vi "LINC Register Commit.vi"(4 "override? registration":bool, 8 "error in (no error)":errorcluster, 10 "register":T1={"COSMOS cmds (T)"=TRUE, "common cmds (T)"=TRUE, "handshake tlm (T)"=TRUE, "error tlm (T)"=TRUE}, 11 "LINC session":refnum<class "LINC.lvclass">) -> (0 "error out":errorcluster, 3 "dup LINC session":refnum<class "LINC.lvclass">)   [LabVIEW 2018, in "STEPkgDriver_LINC.lvlib" / "LINC.lvclass"]
uses:
  LINC.lvclass
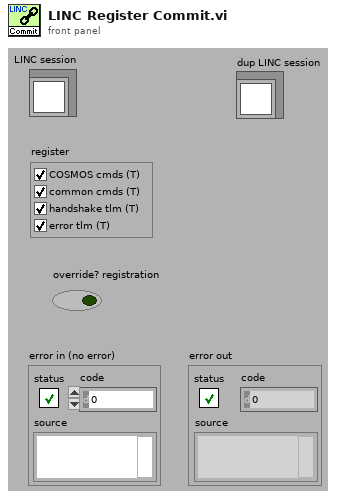
[diagram p1: front panel]
types:
  T1 = cluster{"COSMOS cmds (T)":bool, "common cmds (T)":bool, "handshake tlm (T)":bool, "error tlm (T)":bool}
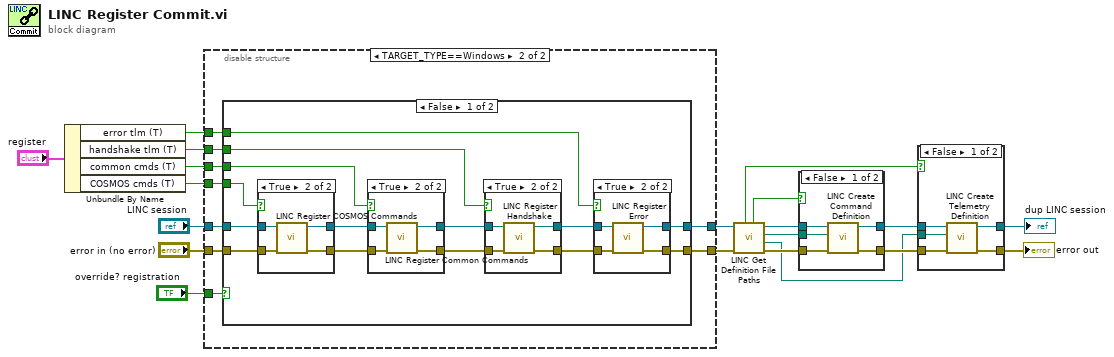
[diagram p0: block diagram]
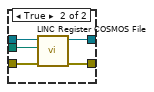
[diagram p8: hidden frame]
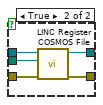
[diagram p9: hidden frame]
diagram:
  n1 = Unbundle By Name("register") -> ("error tlm (T)"=w5:bool, "handshake tlm (T)"=w2:bool, "common cmds (T)"=w3:bool, "COSMOS cmds (T)"=w4:bool)
  n2 = disable-structure shown="TARGET_TYPE==Windows" {
    disable-tunnel: "error in (no error)" -> [w21 w30]
    disable-tunnel: "LINC session" -> [w22 w29]
    disable-tunnel: [w21 w24] -> w16
    disable-tunnel: [w22 w25] -> w7
    disable-tunnel: w3 -> [_ w31]
    disable-tunnel: w5 -> [_ w26]
    disable-tunnel: w4 -> [_ w28]
    disable-tunnel: w2 -> [_ w27]
    disable-tunnel: "override? registration" -> [_ w23]
    frame condition #0 {
      # "Dynamic Registration is not available in any target type but Windows"
    }
    frame condition #1 (active) {
      n3 = case shown="False" w23 {
        tunnel: w31 -> [w45 _]
        tunnel: w30 -> [w44 w70]
        tunnel: w29 -> [w43 w71]
        tunnel: w28 -> [w40 _]
        tunnel: w27 -> [w37 _]
        tunnel: w26 -> [w34 _]
        tunnel: [w33 w71] -> w25
        tunnel: [w32 w70] -> w24
        frame False {
          n4 = case shown="True" w40 {
            tunnel: w44 -> [w58 w63]
            tunnel: w43 -> [w59 w62]
            tunnel: [w58 w61] -> w41
            tunnel: [w59 w60] -> w42
            frame False {
            }
            frame True {
              n5 = call "LINC Register COSMOS Commands.vi"("error in"=w63, "LINC session"=w62) -> ("error out"=w61:errorcluster, "dup LINC session"=w60:refnum<class "LINC.lvclass">)  [unwired: 8 in]
            }
          }
          n6 = case shown="True" w45 {
            tunnel: w41 -> [w65 w69]
            tunnel: [w65 w68] -> w38
            tunnel: [w64 w67] -> w39
            tunnel: w42 -> [w64 w66]
            frame False {
            }
            frame True {
              n7 = call "LINC Register Common Commands.vi"("error in"=w69, "LINC session"=w66) -> ("error out"=w68:errorcluster, "dup LINC session"=w67:refnum<class "LINC.lvclass">)  [unwired: 8 in]
            }
          }
          n8 = case shown="True" w37 {
            tunnel: w38 -> [w53 w57]
            tunnel: [w53 w56] -> w36
            tunnel: [w52 w55] -> w35
            tunnel: w39 -> [w52 w54]
            frame False {
            }
            frame True {
              n9 = call "LINC Register Handshake.vi"("error in (no error)"=w57, "LINC session"=w54) -> ("error out"=w56:errorcluster, "dup LINC session"=w55:refnum<class "LINC.lvclass">)  [unwired: 8 in]
            }
          }
          n10 = case shown="True" w34 {
            tunnel: w36 -> [w47 w51]
            tunnel: [w47 w50] -> w32
            tunnel: [w46 w49] -> w33
            tunnel: w35 -> [w46 w48]
            frame False {
            }
            frame True {
              n11 = call "LINC Register Error.vi"("error in (no error)"=w51, "LINC session"=w48) -> ("error out"=w50:errorcluster, "dup LINC session"=w49:refnum<class "LINC.lvclass">)  [unwired: 8 in]
            }
          }
        }
        frame True {
        }
      }
    }
  }
  n12 = call "LINC Get Definition File Paths.vi"("error in (no error)"=w16, "LINC session"=w7) -> ("error out"=w15:errorcluster, "TLM defintion path"=w13:path, "CMD definition path"=w14:path, "dup LINC session"=w12:refnum<class "LINC.lvclass">, "CMD definition exists"=w11:bool, "TLM definition exists"=w10:bool)  [unwired: 4 in]
  n13 = case shown="False" w11 {
    tunnel: [w76 w78] -> w20
    tunnel: [w75 w77] -> w19
    tunnel: w15 -> [w74 w81]
    tunnel: w12 -> [w73 w80]
    tunnel: w14 -> [w72 w79]
    frame False {
      n14 = call "LINC Create Command Definition.vi"("error in (no error)"=w74, "path"=w72, "LINC session"=w73) -> ("error out"=w75:errorcluster, "dup LINC session"=w76:refnum<class "LINC.lvclass">)  [unwired: 7 in]
    }
    frame True {
      n15 = call "LINC Register COSMOS File.vi"("error in (no error)"=w81, "path"=w79, "LINC session"=w80) -> ("error out"=w77:errorcluster, "dup LINC session"=w78:refnum<class "LINC.lvclass">)  [unwired: 7 in]
    }
  }
  n16 = case shown="False" w10 {
    tunnel: w20 -> [w86 w90]
    tunnel: w19 -> [w85 w91]
    tunnel: [w84 w89] -> w9
    tunnel: [w83 w88] -> w8
    tunnel: w13 -> [w82 w87]
    frame False {
      n17 = call "LINC Create Telemetry Definition.vi"("error in (no error)"=w85, "path"=w82, "LINC session"=w86) -> ("error out"=w83:errorcluster, "dup LINC session"=w84:refnum<class "LINC.lvclass">)  [unwired: 7 in]
    }
    frame True {
      n18 = call "LINC Register COSMOS File.vi"("error in (no error)"=w91, "path"=w87, "LINC session"=w90) -> ("error out"=w88:errorcluster, "dup LINC session"=w89:refnum<class "LINC.lvclass">)  [unwired: 7 in]
    }
  }
  "error out" <- w8
  "dup LINC session" <- w9
